vi "PathPlanner_FieldUtil_FlipFieldPosition.vi"(11 "FieldPosition":T1={"X"=0.0, "Y"=1.0} {"Y" format="%14.3f"; "X" format="%14.3f"}) -> (3 "FlippedFieldPosition":T1={"X"=0.0, "Y"=1.0} {"Y" format="%14.3f"; "X" format="%14.3f"})   [LabVIEW 2019, in "PathPlanner24.lvlib"]
doc: "The X size or length of the current field in meters\n\nInput:\n -- <none>\n\nOutputs:\n -- FieldSizeX -- X length of field (meters)"
uses:
  <vilib>/Rock Robotics/WPI/ThirdParty/JAS_Junk/TrajLib/Rotation2d_UnaryMinus.vi
  <vilib>/Rock Robotics/WPI/ThirdParty/JAS_Junk/TrajLib/Rotation2d_RotateBy.vi
  <vilib>/Rock Robotics/WPI/ThirdParty/JAS_Junk/TrajLib/Rotation2d_CreateXY.vi
  <vilib>/Rock Robotics/WPI/ThirdParty/JAS_Junk/TrajLib/Util_CalcDist.vi
  PathPlanner24.lvlib
  <vilib>/Rock Robotics/WPI/ThirdParty/JAS_Junk/TrajLib/Trajectory_Library.lvlib
  <vilib>/Rock Robotics/WPI/ThirdParty/JAS_Junk/TrajLib/TypeDef/TRANSLATION2D.ctl
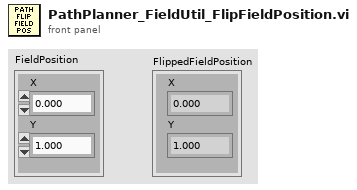
[diagram p1: front panel]
types:
  T1 = typedef "Trajectory_Library.lvlib/TRANSLATION2D.ctl" = cluster{"X":dbl, "Y":dbl}
  T2 = typedef "PathPlanner24.lvlib/PathPlanner_FieldSymmetry_ENUM.ctl" = enum16{"kRotational", "kMirrored"}
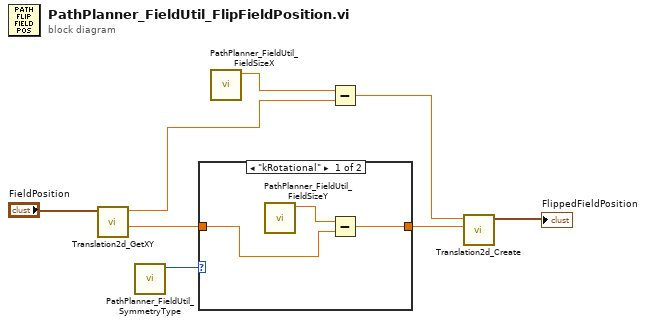
[diagram p0: block diagram]
diagram:
  n1 = call <vilib>:"Translation2d_GetXY.vi"("In Translation"="FieldPosition") -> ("Y"=w5:dbl, "X"=w2:dbl)  [unwired: 9 in]
  n2 = call "PathPlanner_FieldUtil_SymmetryType.vi"() -> ("PathPlanner_FieldSymmetry"=w8:T2)  [unwired: 11 in]
  n3 = case shown="\"kRotational\"" w8 {
    tunnel: w5 -> [w10 w12]
    tunnel: [w9 w12] -> w4
    frame "kRotational" {
      n4 = call "PathPlanner_FieldUtil_FieldSizeY.vi"() -> ("FieldSizeY_M"=w11:dbl)  [unwired: 11 in]
      n5 = Subtract(x=w11, y=w10) -> (x-y=w9:dbl)
    }
    frame "kMirrored" {
    }
  }
  n6 = call "PathPlanner_FieldUtil_FieldSizeX.vi"() -> ("FieldSizeX_M"=w3:dbl)  [unwired: 11 in]
  n7 = Subtract(x=w3, y=w2) -> (x-y=w1:dbl)
  n8 = call <vilib>:"Translation2d_Create.vi"("Y"=w4, "X"=w1) -> ("TRANSLATION"=→"FlippedFieldPosition":T1)  [unwired: 9 in]
